vi "Get Time.vi"(0 "t_high":u32[](array[numeric]), 5 "t_low":u32[](array[numeric]), 7 "Start Time (s)":dbl, 9 "Time Base (s)":sgl format="%#_13g", 11 "error in (no error)":errorcluster) -> (8 "Time":dbl[](array[numeric]), 15 "error out":errorcluster)   [LabVIEW 2018, in "Potentiostat Galvanostat.lvclass"]
doc: "This function tests the communication speed between the library and the selected channel. \nNOTE: This function is for advanced user only."
uses:
  Potentiostat Galvanostat.lvclass
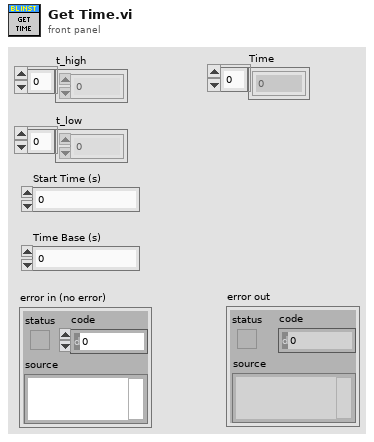
[diagram p1: front panel]
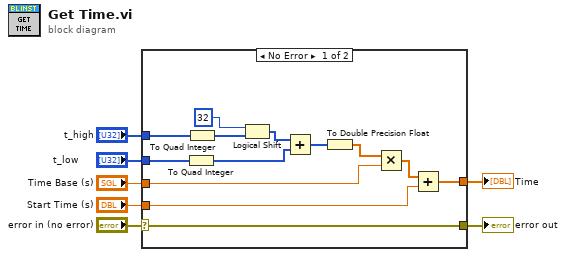
[diagram p0: block diagram]
diagram:
  n1 = case shown="No Error" "error in (no error)" {
    selector: "error in (no error)" -> [w20 w21]
    tunnel: [w20 w21] -> w7
    tunnel: "Start Time (s)" -> [w13 _]
    tunnel: "Time Base (s)" -> [w15 _]
    tunnel: "t_high" -> [w19 _]
    tunnel: "t_low" -> [w18 _]
    tunnel: [w11 _] -> w1
    frame No Error {
      n2 = To Quad Integer(1:w18) -> (0:w17:i64[])
      n3 = To Quad Integer(1:w19) -> (0:w9:i64[])
      n4 = Logical Shift(y=i16 32, x=w9) -> (x << y=w8:i64[])
      n5 = Add(x=w8, y=w17) -> (x+y=w16:i64[])
      n6 = To Double Precision Float(number=w16) -> (double precision float=w14:dbl[])
      n7 = Multiply(x=w14, y=w15) -> (x*y=w12:dbl[])
      n8 = Add(x=w12, y=w13) -> (x+y=w11:dbl[])
    }
    frame Error {
    }
  }
  "error out" <- w7
  "Time" <- w1
